vi "读取数据属性.vi"(11 "测试数据":T1) -> (3 "数据属性":string[][](array[string]))   [LabVIEW 2020]
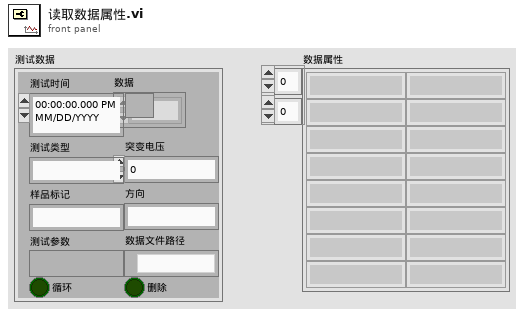
[diagram p1: front panel]
types:
  T1 = typedef "测试数据类型.ctl" = cluster{"测试时间":timestamp, "测试类型":string, "样品标记":string, "测试参数":variant, "循环":bool, "数据":dbl[][], "删除":bool, "突变电压":i32, "方向":string, "数据文件路径":path}
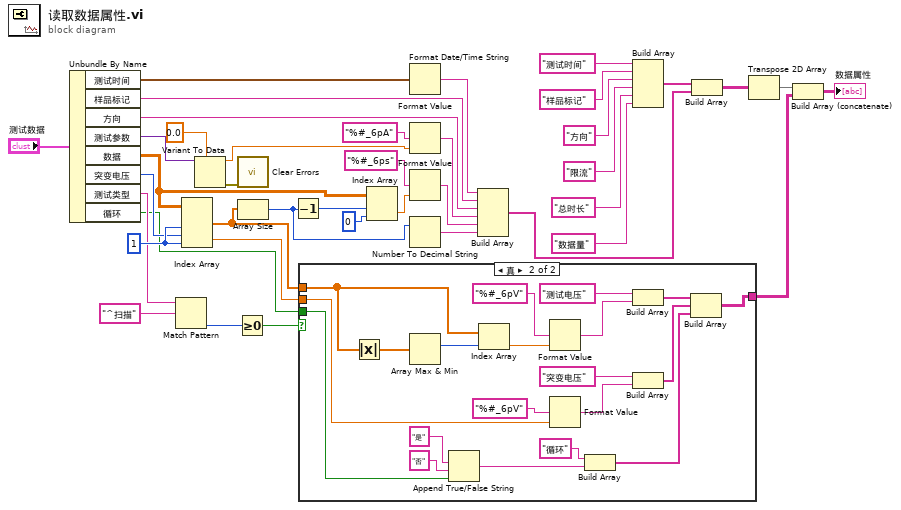
[diagram p0: block diagram]
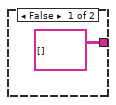
[diagram p2: hidden frame]
diagram:
  w8 = 1 ("索引 (列)")
  n1 = Unbundle By Name("测试数据") -> ("测试时间"=w26:timestamp, "样品标记"=w29:string, "方向"=w30:string, "测试参数"=w31:variant, "数据"=w15:dbl[][], "突变电压"=w7:i32, "测试类型"=w3:string, "循环"=w2:bool)
  n2 = Match Pattern(string=w3, regular expression="^扫描" ("字符串")) -> (offset past match=w21:i32)  [unwired: 1 in, 3 out]
  n3 = Index Array(array=w15, index (col) #1=w8, index (row) #2=w7, index (col) #2=w8) -> (element #1=w5:dbl[], element #2=w6:dbl)  [unwired: 1 in]
  n4 = Variant To Data(type=0.0, Variant=w31) -> (data=w34:dbl, error out=w1:errorcluster)  [unwired: 1 in]
  n5 = Greater Or Equal To 0?(x=w21) -> (x >= 0?=w20:bool)
  n6 = call <vilib>:"Clear Errors.vi"("error in (no error)"=w1) -> ()  [unwired: 5 in, 2 out]
  n7 = Array Size(array=w5) -> (size(s)=w4:i32)
  n8 = Decrement(x=w4) -> (x-1=w14:i32)
  n9 = case shown="真" w20 {
    tunnel: [string[][] [] ("数组") w55] -> w18
    tunnel: w2 -> [_ w48]
    tunnel: w5 -> [_ w44]
    tunnel: w6 -> [_ w47]
    frame False {
    }
    frame True {
      n10 = Absolute Value(x=w44) -> (abs(x)=w45:dbl[])
      n11 = Array Max & Min(array=w45) -> (max index (indices)=w43:i32)  [unwired: 3 out]
      n12 = Append True/False String(1:w48, 2:"否" ("假字符串"), 3:"是" ("真字符串")) -> (0:w58:string)  [unwired: 1 in]
      n13 = Index Array(array=w44, index=w43) -> (element=w42:dbl)
      n14 = Format Value(format string="%#_6pV" ("格式字符串"), value (0)=w42) -> (output string=w53:string)  [unwired: 1 in]
      n15 = Format Value(format string="%#_6pV" ("格式字符串"), value (0)=w47) -> (output string=w51:string)  [unwired: 1 in]
      n16 = Build Array("循环" ("元素"), w58) -> (w46:string[])
      n17 = Build Array("测试电压" ("元素"), w53) -> (w56:string[])
      n18 = Build Array("突变电压" ("元素"), w51) -> (w49:string[])
      n19 = Build Array(w56, w49, w46) -> (w55:string[][])
    }
  }
  n20 = Index Array(array=w15, index (row)=w14, index (col)=0 ("禁用的索引 (列)")) -> (element=w12:dbl)
  n21 = Format Date/Time String(seconds (now)=w26) -> (date/time string=w27:string)  [unwired: 2 in]
  n22 = Format Value(format string="%#_6pA" ("格式字符串"), value (0)=w34) -> (output string=w36:string)  [unwired: 1 in]
  n23 = Format Value(format string="%#_6ps" ("格式字符串"), value (0)=w12) -> (output string=w11:string)  [unwired: 1 in]
  n24 = Number To Decimal String(number=w4) -> (decimal integer string=w9:string)  [unwired: 1 in]
  n25 = Build Array(w27, w29, w30, w36, w11, w9) -> (w38:string[])
  n26 = Build Array("测试时间" ("日期/时间字符串"), "样品标记" ("元素"), "方向" ("元素"), "限流" ("元素"), "总时长" ("元素"), "数据量" ("元素")) -> (w37:string[])
  n27 = Build Array(w37, w38) -> (w39:string[][])
  n28 = Transpose 2D Array(2D array=w39) -> (transposed array=w40:string[][])
  n29 = Build Array (concatenate)(w40, w18) -> (→"数据属性":string[][])
